vi "Load Config.vi"(8 "error in (no error)":errorcluster, 9 "Timeout mS (30000)":i32=30000, 11 "ConfigAPI in":refnum<class "ConfigAPI.lvclass">) -> (0 "error out":errorcluster, 2 "Node":refnum<class "Node.lvclass">, 3 "ConfigAPI out":refnum<class "ConfigAPI.lvclass">)   [LabVIEW 2020, in "Volatus.lvlib" / "ConfigAPI.lvclass"]
uses:
  ConfigAPI.lvclass
  ConfigAPI.lvclass/ConfigAPI.ctl
  VolatusConfigManager Messages/Load Config Msg/Load Config Msg.lvclass
  lv-promises/Promises/Promise/Promise.lvclass
  VolatusNodeValue/VolatusNodeValue.lvclass
  lv-promises/Promises/Future/Future.lvclass
  C:/dev/lv20CE/relink/lv-promises/Promises/Value/Value.lvclass
  C:/dev/lv20CE/relink/lv-volatus/Volatus/VolatusNodeValue/VolatusNodeValue.lvclass
  VolatusConfig/Node/Node.lvclass
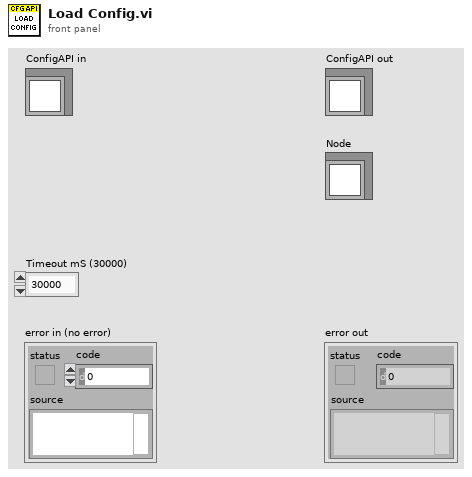
[diagram p1: front panel]
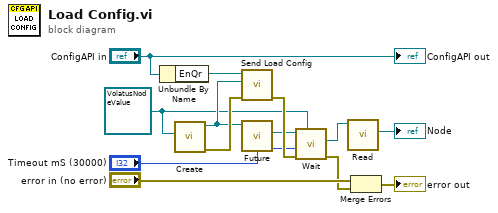
[diagram p0: block diagram]
diagram:
  w5 = refnum<class "VolatusNodeValue.lvclass"> refnum ("Volatus:VolatusNodeValue.lvclass")
  n1 = Unbundle By Name("ConfigAPI in") -> ("EnQr"=w10:refnum<class "Message Enqueuer.lvclass">)
  n2 = call "Create.vi"("Result Type"=w5) -> ("error out"=w9:errorcluster, "Promise"=w8:refnum<class "Promise.lvclass">)  [unwired: 9 in]
  n3 = call "Send Load Config.vi"("error in (no error)"=w9, "Promise"=w8, "Message Enqueuer"=w10) -> ("error out"=w13:errorcluster)  [unwired: 7 in, 1 out]
  n4 = call "Future.vi"("Promise in"=w8) -> ("Future"=w7:refnum<class "Future.lvclass">)  [unwired: 9 in, 1 out]
  n5 = call "Wait.vi"("Result Type"=w5, "error in (no error)"=w13, "Timeout mS (-1)"="Timeout mS (30000)", "Future in"=w7) -> ("error out"=w2:errorcluster, "Result"=w4:refnum<class "VolatusNodeValue.lvclass">)  [unwired: 6 in]
  n6 = call "Read.vi"("VolatusNodeValue in"=w4) -> ("Node"=→"Node":refnum<class "Node.lvclass">)  [unwired: 10 in]
  n7 = Merge Errors("error in (no error)", w2) -> (→"error out":errorcluster)
  "ConfigAPI out" <- "ConfigAPI in"
